vi "template-state-machine-iwh.vi"() -> ()   [LabVIEW 2024]
uses:
  state-enum.ctl
  csv-file-logging/filepath-selection.ctl
  csv-file-logging/datalogging-options.ctl
  serial-options.ctl
  sensor-options.ctl
panel:
  out "Serial Port Open":bool
  out "return count":u32
  out "Bytes at Port":u32
  out "Log File Open":bool
  in  "Tab Control":enum32{"Data", "Settings"}(tab)
  out "Units":string
  out "Data":dbl
  out "Data Plot Chart":dbl(graph)
  out "Logged CSV out":string
  out "Serial msg":string
  in  "Datalogging options":T1={"data-precision"=3, "Include Date"=FALSE, "Include Timestamp"=TRUE, "Include Milliseconds"=FALSE, "sample-rate (Hz)"=4.0}
  in  "Log Filepath Selection":T2={"Log Filepath Source"=enum."Application Relative (Auto)", "Log File Path (Manual)"=path "C:/Users/dheard/Documents/0002-labview-projects/adam-4xxx/template/data", "Log File Folder Name"="data", "log file name"="log", "Include Date in Filename"=TRUE, "Include Time in Filename"=TRUE}
  in  "Serial Port Options":T3={"COM Port (COM10)"="COM10", "baud rate (19200)"=19200} {"baud rate (19200)" max=115200 step=1200}
  in  "Sensor Options":T4={"Display Units"="log", "Zero Offset"=2.62, "Sensor Min"=0.0, "Sensor Max"=500.0, "Signal Min"=0.0, "Signal Max"=100.0, "Conversion Factor"=0.0}
  out "Sample Rate (Hz)":dbl format="%-#3.3f"
  in  "Debug Mode":bool
  out "Loop Time (mS)":u32
  out "State:":T5
  out "error IO":errorcluster
  in  "stop":bool
  in  "start":bool
  in  "Exit":bool
  # "Template State Machine"
  # "1. Units of Data: The data will be in PSI (pounds per square inch).\n2. Sample Rate Required: The required sample rate is 4 Hz (each 0.25 seconds)\n3. Data Display: The data should be displayed in real-time as a graphical chart with numerical values.\n4. Logging Requirements:\n   - We need to log all data.\n   - The preferred formats are CSV and Excel.\n   - Data should be timestamped with a standard date and time format (e.g., YYYY-MM-DD HH:MM:SS).\n \n5. Data Format: Attached is a sample of the expected data with the correct formatting to guide the reproduction process."
  # "Live Data"
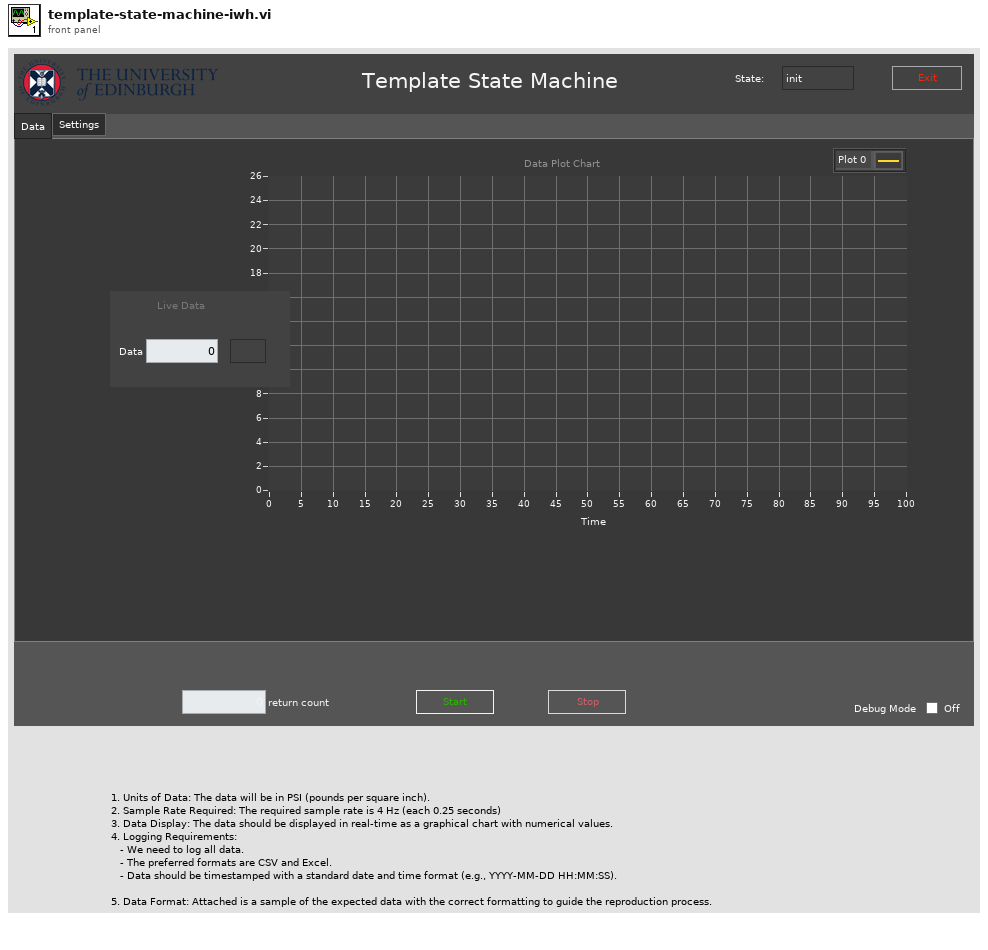
[diagram p1: front panel]
types:
  T1 = typedef "datalogging-options.ctl" = cluster{"data-precision":i32, "Include Date":bool, "Include Timestamp":bool, "Include Milliseconds":bool, "sample-rate (Hz)":dbl}
  T2 = typedef "filepath-selection.ctl" = cluster{"Log Filepath Source":enum16{"Application Relative (Auto)", "VI Relative (Auto)", "Complete Path (Manual)"}, "Log File Path (Manual)":path, "Log File Folder Name":string, "log file name":string, "Include Date in Filename":bool, "Include Time in Filename":bool}
  T3 = typedef "serial-options.ctl" = cluster{"COM Port (COM10)":refnum<visa-resource-name>, "baud rate (19200)":u32}
  T4 = typedef "sensor-options.ctl" = cluster{"Display Units":string, "Zero Offset":dbl, "Sensor Min":dbl, "Sensor Max":dbl, "Signal Min":dbl, "Signal Max":dbl, "Conversion Factor":dbl}
  T5 = typedef "state-enum.ctl" = enum16{"init", "wait", "start", "run", "stop", "shutdown", "exit"}
  T6 = enum8{"Enabled", "Disabled", "Disabled and Grayed Out"}
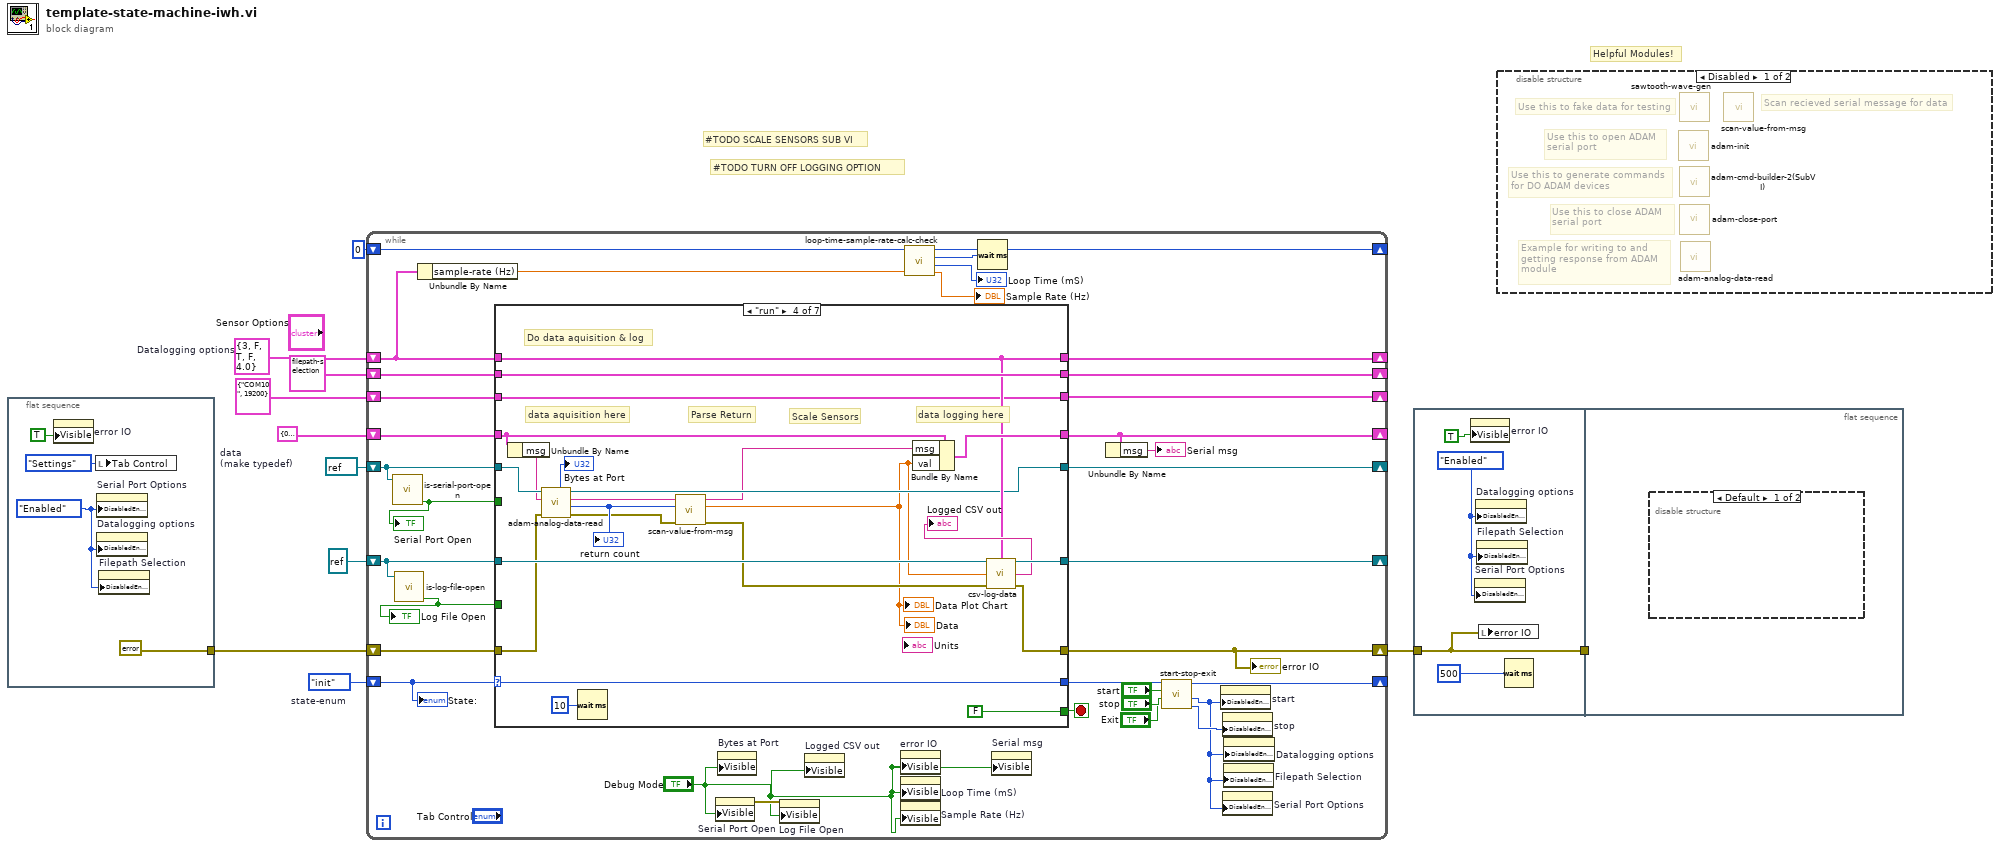
[diagram p0: block diagram]
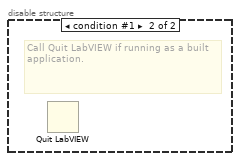
[diagram p3: hidden frame]
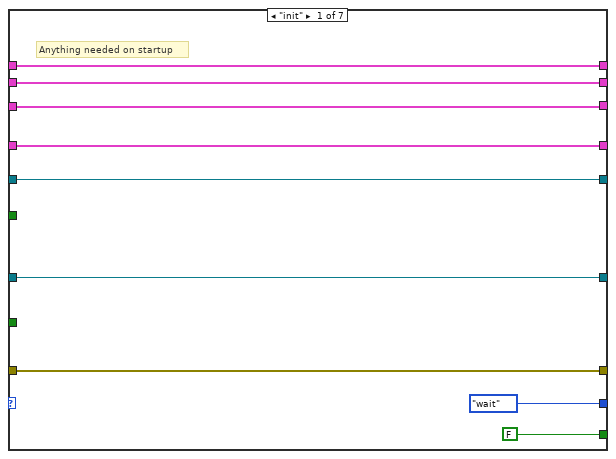
[diagram p4: hidden frame]
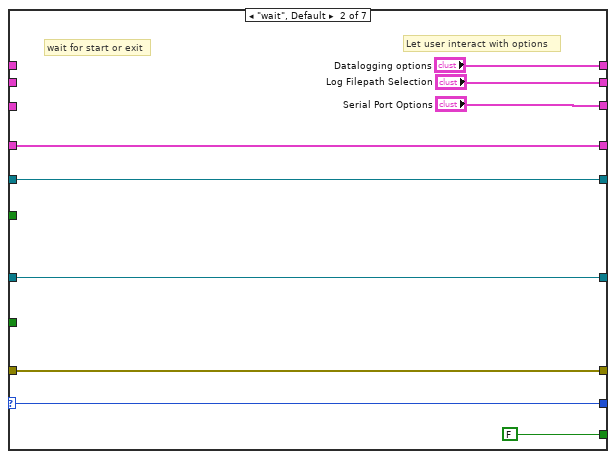
[diagram p5: hidden frame]
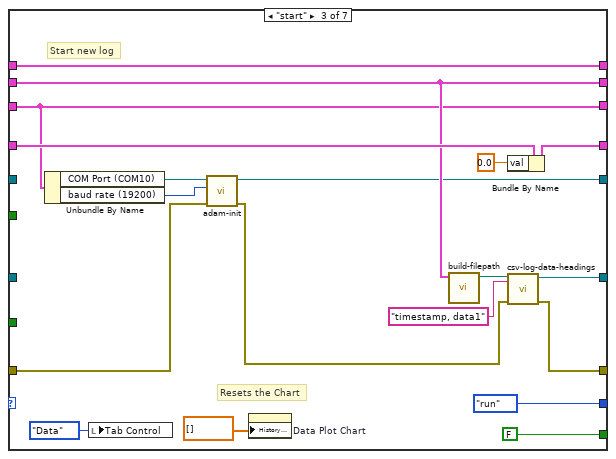
[diagram p6: hidden frame]
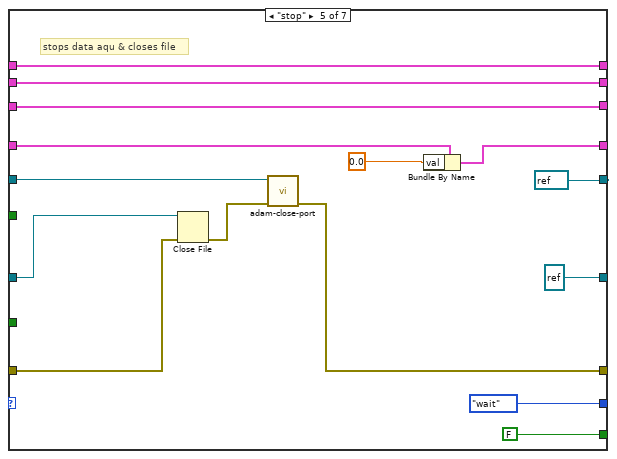
[diagram p7: hidden frame]
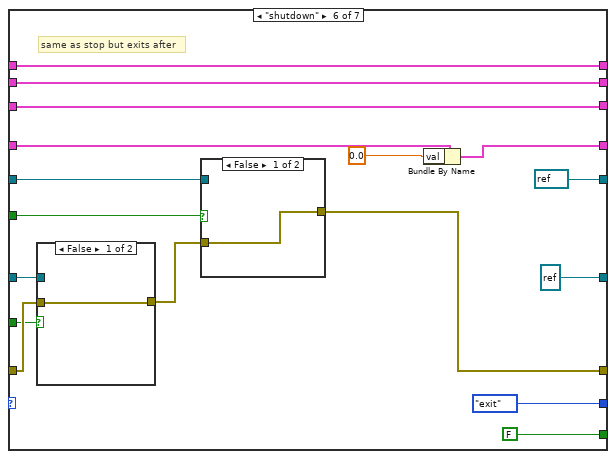
[diagram p8: hidden frame]
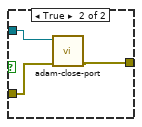
[diagram p9: hidden frame]
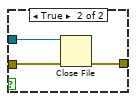
[diagram p10: hidden frame]
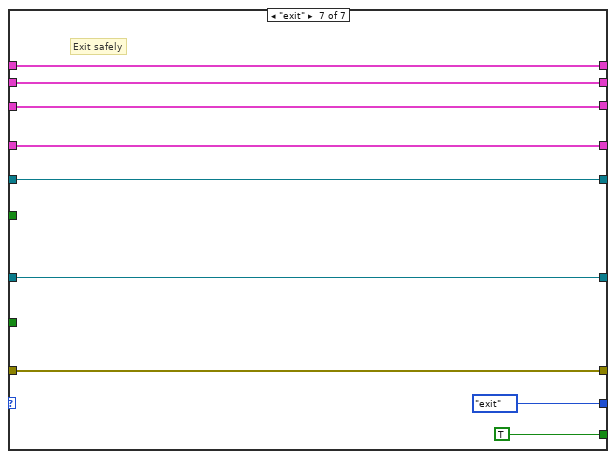
[diagram p11: hidden frame]
diagram:
  w3 = T1 {"data-precision"=3, "Include Date"=FALSE, "Include Timestamp"=TRUE, "Include Milliseconds"=FALSE, "sample-rate (Hz)"=4.0}  # Datalogging options
  w8 = cluster{"val":dbl, "bool":bool, "msg":string} {"val"=0.0, "bool"=FALSE, "msg"=""}  # data (make typedef)
  w11 = state-enum."init"  # state-enum
  # "#TODO TURN OFF LOGGING OPTION"
  # "#TODO SCALE SENSORS SUB VI"
  # "Helpful Modules!"
  n1 = flat-sequence {
    tunnel: [errorcluster {"status"=FALSE, "code"=0, "source"=""} ("error IO")] -> w7
    frame #0 {
      w12 = T6."Enabled" ("Disabled")
      n2 = property on="error IO" class="Clust (strict)"("Visible"=TRUE) -> ()  [unwired: 2 in, 2 out]
      n3 = local write "Tab Control"(enum32{"Data", "Settings"}."Settings" ("Tab Control")) -> ()
      n4 = property on="Serial Port Options" class="Clust (strict)"("DisabledEnum"=w12) -> ()  [unwired: 2 in, 2 out]
      n5 = property on="Datalogging options" class="Clust (strict)"("DisabledEnum"=w12) -> ()  [unwired: 2 in, 2 out]
      n6 = property on="Filepath Selection" class="Clust (strict)"("DisabledEnum"=w12) -> ()  [unwired: 2 in, 2 out]
    }
  }
  n7 = while {
    shift-right: [w47] -> _
    shift-left: w11 -> [w49]
    shift-right: [w41] -> w9
    shift-left: w7 -> [w42]
    shift-right: [w19] -> _
    shift-left: w8 -> [w40]
    shift-right: [w37] -> _
    shift-left: u32 0 ("millisecond timer value") -> [w39]
    shift-right: [w33] -> _
    shift-left: T2 {"Log Filepath Source"=enum."Application Relative (Auto)", "Log File Path (Manual)"=path "C:/Users/dheard/Documents/0002-labview-projects/ammonia-absorbsion-rig/data", "Log File Folder Name"="data", "log file name"="log", "Include Date in Filename"=TRUE, "Include Time in Filename"=TRUE} ("Filepath Selection") -> [w32]
    shift-right: [w31] -> _
    shift-left: refnum<file> refnum ("Byte Stream File out") -> [w29]
    shift-right: [w30] -> _
    shift-left: w3 -> [w27]
    shift-right: [w24] -> _
    shift-left: T3 {"COM Port (COM10)"="COM10", "baud rate (19200)"=19200} ("Serial Port Options") -> [w25]
    shift-right: [w22] -> _
    shift-left: refnum<visa-resource-name> refnum ("VISA resource name out") -> [w21]
    stop <- w43 stop-if-true
    n8 = call "is-serial-port-open.vi"("VISA Refnum in"=w21) -> ("port-status"=w16:bool)  [unwired: 10 in]
    "Serial Port Open" <- w16
    n9 = call "is-log-file-open.vi"("Byte Stream File in"=w29) -> ("Log File Open"=w28:bool)  [unwired: 10 in]
    "Log File Open" <- w28
    n10 = Unbundle By Name(w27) -> ("sample-rate (Hz)"=w26:dbl)
    n11 = case shown="\"run\"" w49 {
      selector: w49 -> [_ w67 _ w108 _ _ _]
      tunnel: [state-enum."wait" w67 state-enum."run" w108 state-enum."wait" state-enum."exit" state-enum."exit"] -> w48
      tunnel: [FALSE FALSE FALSE FALSE FALSE FALSE TRUE] -> w43
      tunnel: [w56 w65 w76 w102 w110 w125 w156] -> w41
      tunnel: w42 -> [w56 w65 w69 w98 w117 w134 w156]
      tunnel: [w55 w64 w83 w107 w120 w137 w155] -> w19
      tunnel: w40 -> [w55 w64 w84 w94 w122 w139 w155]
      tunnel: [w53 "Log Filepath Selection" w80 w103 w116 w133 w153] -> w33
      tunnel: w32 -> [w53 _ w80 w103 w116 w133 w153]
      tunnel: [w54 w62 w77 w105 refnum<file> refnum ("log file Byte Stream File out") refnum<file> refnum ("log file Byte Stream File out") w154] -> w31
      tunnel: w29 -> [w54 w62 _ w106 w119 w136 w154]
      tunnel: [w52 "Datalogging options" w74 w101 w115 w132 w152] -> w30
      tunnel: w27 -> [w52 _ w74 w101 w115 w132 w152]
      tunnel: w28 -> [_ _ _ _ _ w131 _]
      tunnel: w25 -> [w51 _ w73 w100 w114 w130 w151]
      tunnel: [w51 "Serial Port Options" w73 w100 w114 w130 w151] -> w24
      tunnel: [w50 w59 w70 w96 refnum<visa-resource-name> refnum ("VISA resource name out") refnum<visa-resource-name> refnum ("VISA resource name out") w150] -> w22
      tunnel: w21 -> [w50 w59 _ w99 w113 w128 w150]
      tunnel: w16 -> [_ _ _ _ _ w129 _]
      frame "init" {
        # "Anything needed on startup"
      }
      frame "wait", Default {
        # "Let user interact with options"
        # "wait for start or exit"
      }
      frame "start" {
        # "Start new log"
        # "Resets the Chart"
        n12 = Unbundle By Name(w73) -> ("COM Port (COM10)"=w72:refnum<visa-resource-name>, "baud rate (19200)"=w71:u32)
        n13 = local write "Tab Control"(enum32{"Data", "Settings"}."Data" ("Tab Control")) -> ()
        n14 = call "adam-init.vi"("error in (no error)"=w69, "baud rate (19200)"=w71, "COM Port (COM10)"=w72) -> ("error out"=w68:errorcluster, "VISA resource name out"=w70:refnum<visa-resource-name>)  [unwired: 7 in]
        n15 = property on="Data Plot Chart" class="WFChart (strict)"("History Data"=dbl[] []) -> ()  [unwired: 2 in, 2 out]
        n16 = call "build-filepath.vi"("Filepath Selection"=w80) -> ("appended path for log file"=w79:path)  [unwired: 9 in, 1 out]
        n17 = Bundle By Name(cluster=w84, "val"=0.0 ("output")) -> (w83:cluster{"val":dbl, "bool":bool, "msg":string})
        n18 = call "csv-log-data-headings.vi"("CSV Data Headings"="timestamp, data1", "error in (no error)"=w68, "Log File Path"=w79) -> ("error out"=w76:errorcluster, "Byte Stream File out"=w77:refnum<file>)  [unwired: 6 in, 1 out]
      }
      frame "run" {
        # "Scale Sensors"
        # "Parse Return"
        # "data logging here"
        # "data aquisition here"
        # "Do data aquisition & log"
        n19 = Unbundle By Name(w94) -> ("msg"=w93:string)
        n20 = call "adam-analog-data-read.vi"("error in (no error)"=w98, "current-buffer"=w93, "VISA Refnum in"=w99) -> ("error out"=w91:errorcluster, "return count"=w92:u32, "read buffer"=w89:string, "VISA Refnum Out"=w96:refnum<visa-resource-name>, "Bytes at Port"=→"Bytes at Port":u32)  [unwired: 4 in]
        "return count" <- w92
        n21 = Wait (ms)(milliseconds to wait=u32 10) -> ()  [unwired: 1 out]
        n22 = call "scan-value-from-msg.vi"("error in (no error)"=w91, "msg length"=w92, "read buffer in"=w89) -> ("error out"=w90:errorcluster, "Raw Data"=w87:dbl, "read buffer out"=w88:string)  [unwired: 6 in]
        "Data" <- w87
        "Data Plot Chart" <- w87
        n23 = Bundle By Name(cluster=w94, "msg"=w88, "val"=w87) -> (w107:cluster{"val":dbl, "bool":bool, "msg":string})
        n24 = call "csv-log-data.vi"("log file Byte Stream File in"=w106, "Datalogging options"=w101, "Data Point In"=w87, "error in (no error)"=w90) -> ("log file Byte Stream File out"=w105:refnum<file>, "Logged CSV out"=→"Logged CSV out":string, "error out"=w102:errorcluster)  [unwired: 7 in, 2 out]
      }
      frame "stop" {
        # "stops data aqu & closes file"
        n25 = Close File(refnum=w119, error in=w117) -> (error out=w111:errorcluster)  [unwired: 1 out]
        n26 = call "adam-close-port.vi"("error in (no error)"=w111, "VISA Refnum in"=w113) -> ("error out"=w110:errorcluster)  [unwired: 9 in]
        n27 = Bundle By Name(cluster=w122, "val"=0.0 ("output")) -> (w120:cluster{"val":dbl, "bool":bool, "msg":string})
      }
      frame "shutdown" {
        # "same as stop but exits after"
        n28 = case shown="False" w131 {
          tunnel: w136 -> [_ w149]
          tunnel: w134 -> [w146 w148]
          tunnel: [w146 w147] -> w126
          frame False {
          }
          frame True {
            n29 = Close File(refnum=w149, error in=w148) -> (error out=w147:errorcluster)  [unwired: 1 out]
          }
        }
        n30 = case shown="False" w129 {
          tunnel: w128 -> [_ w145]
          tunnel: w126 -> [w142 w144]
          tunnel: [w142 w143] -> w125
          frame False {
          }
          frame True {
            n31 = call "adam-close-port.vi"("error in (no error)"=w144, "VISA Refnum in"=w145) -> ("error out"=w143:errorcluster)  [unwired: 9 in]
          }
        }
        n32 = Bundle By Name(cluster=w139, "val"=0.0 ("output")) -> (w137:cluster{"val":dbl, "bool":bool, "msg":string})
      }
      frame "exit" {
        # "Exit safely"
      }
    }
    "error IO" <- w41
    n33 = property on="Serial Port Open" class="Bool (strict)"("Visible"="Debug Mode") -> (error out=w20:errorcluster)  [unwired: 2 in, 1 out]
    n34 = property on="Bytes at Port" class="DigNum (strict)"("Visible"="Debug Mode") -> ()  [unwired: 2 in, 2 out]
    n35 = property on="Log File Open" class="Bool (strict)"(error in=w20, "Visible"="Debug Mode") -> ()  [unwired: 1 in, 2 out]
    n36 = property on="Logged CSV out" class="Str"("Visible"="Debug Mode") -> ()  [unwired: 2 in, 2 out]
    n37 = property on="error IO" class="Clust (strict)"("Visible"="Debug Mode") -> ()  [unwired: 2 in, 2 out]
    n38 = property on="Loop Time (mS)" class="DigNum (strict)"("Visible"="Debug Mode") -> ()  [unwired: 2 in, 2 out]
    n39 = property on="Sample Rate (Hz)" class="DigNum (strict)"("Visible"="Debug Mode") -> ()  [unwired: 2 in, 2 out]
    n40 = call "loop-time-sample-rate-calc-check.vi"("sample-rate-Hz"=w26, "millisecond timer value in"=w39) -> ("Loop Hz"=→"Sample Rate (Hz)":dbl, "Loop Time (mS)"=→"Loop Time (mS)":u32, "sample-rate-delay-mS"=w34:u32, "millisecond timer value out"=w37:u32)  [unwired: 6 in]
    n41 = Wait (ms)(milliseconds to wait=w34) -> ()  [unwired: 1 out]
    n42 = property on="Serial msg" class="Str"("Visible"="Debug Mode") -> ()  [unwired: 2 in, 2 out]
    n43 = Unbundle By Name(w19) -> ("msg"=→"Serial msg":string)
    n44 = call "start-stop-exit.vi"("Exit"="Exit", "stop"="stop", "start"="start", "current-state"=w48) -> ("stop-enable"=w38:T6, "start-enable"=w23:T6, "new-state"=w47:T5)  [unwired: 5 in]
    n45 = property on="start" class="Bool"("DisabledEnum"=w23) -> ()  [unwired: 2 in, 2 out]
    n46 = property on="stop" class="Bool"("DisabledEnum"=w38) -> ()  [unwired: 2 in, 2 out]
    n47 = property on="Serial Port Options" class="Clust (strict)"("DisabledEnum"=w23) -> ()  [unwired: 2 in, 2 out]
    n48 = property on="Filepath Selection" class="Clust (strict)"("DisabledEnum"=w23) -> ()  [unwired: 2 in, 2 out]
    n49 = property on="Datalogging options" class="Clust (strict)"("DisabledEnum"=w23) -> ()  [unwired: 2 in, 2 out]
    "State:" <- w49
  }
  n50 = flat-sequence {
    tunnel: [w160] -> w10
    tunnel: w9 -> [w160]
    tunnel: w10 -> [_]
    frame #0 {
      w159 = T6."Enabled" ("Disabled")
      n51 = property on="error IO" class="Clust (strict)"("Visible"=TRUE) -> ()  [unwired: 2 in, 2 out]
      n52 = property on="Serial Port Options" class="Clust (strict)"("DisabledEnum"=w159) -> ()  [unwired: 2 in, 2 out]
      n53 = property on="Datalogging options" class="Clust (strict)"("DisabledEnum"=w159) -> ()  [unwired: 2 in, 2 out]
      n54 = property on="Filepath Selection" class="Clust (strict)"("DisabledEnum"=w159) -> ()  [unwired: 2 in, 2 out]
      n55 = local write "error IO"(w160) -> ()
      n56 = Wait (ms)(milliseconds to wait=u32 500) -> ()  [unwired: 1 out]
    }
    frame #1 {
      n57 = disable-structure "Conditional Disable Structure" shown="Default" {
        frame condition #0 (active) {
        }
        frame condition #1 {
          # "Call Quit LabVIEW if running as a built application."
          n58 = Quit LabVIEW() -> ()  [unwired: 1 in]
        }
      }
    }
  }
  n59 = disable-structure shown="Disabled" {
    frame Disabled {
      # "Scan recieved serial message for data"
      # "Example for writing to and\ngetting response from ADAM\nmodule"
      # "Use this to open ADAM\nserial port"
      # "Use this to close ADAM \nserial port"
      # "Use this to generate commands\nfor DO ADAM devices"
      # "Use this to fake data for testing"
      n60 = call "adam-init.vi"() -> ()  [unwired: 10 in, 2 out]
      n61 = call "sawtooth-wave-gen.vi"() -> ()  [unwired: 11 in, 1 out]
      n62 = call "adam-cmd-builder-2(SubVI).vi"() -> ()  [unwired: 6 in, 6 out]
      n63 = call "adam-close-port.vi"() -> ()  [unwired: 11 in, 1 out]
      n64 = call "adam-analog-data-read.vi"() -> ()  [unwired: 7 in, 5 out]
      n65 = call "scan-value-from-msg.vi"() -> ()  [unwired: 9 in, 3 out]
    }
    frame Enabled {
    }
  }
